vi "myRIOXC Error Strings Global.vi"() -> ()   [LabVIEW 2021]
panel:
  in  "Lengh Not Match Error String":string="The input array length doesn't match the Pins number."
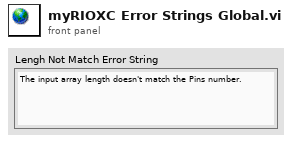
[diagram p1: front panel]
diagram:
